vi "TcpGetDeviceId.vi"(11 "Connection in":T1) -> (2 "DeviceId":string, 3 "Connection out":T1)   [LabVIEW 2017]
uses:
  <vilib>/addons/InsightCM/MessageBus/TcpApi/controls/TcpMessageReference.ctl
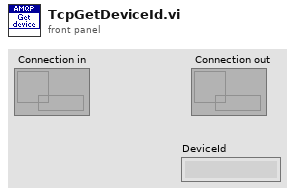
[diagram p1: front panel]
types:
  T1 = typedef "TcpMessageReference.ctl" = refnum<data-value>
  T2 = cluster{"DeviceId":string, "CmdStream":refnum<k5>, "FileStream":refnum<k5>}
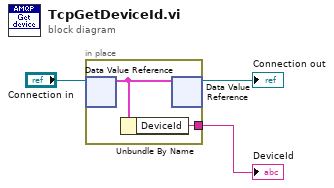
[diagram p0: block diagram]
diagram:
  n1 = in-place {
    in-place-border: [w4] -> w1
    n2 = in-place-dvr #1("Connection in") -> (w5:T2)  [unwired: 1 out]
    n3 = Unbundle By Name(w5) -> ("DeviceId"=w4:string)
    n4 = in-place-dvr #1(w5) -> (→"Connection out":T1)  [unwired: 1 out]
  }
  "DeviceId" <- w1
